vi "WriteIgorDataFile_DP_ver1.0.vi"(2 "2D Data Array In":dbl[][](array[numeric]), 3 "Title Name Array":string[](array[string]), 4 "error in":errorcluster, 5 "Run Info. Comment":string, 7 "file path":path) -> (0 "error out":errorcluster)   [LabVIEW 2012]
doc: "Input 2D data array and Data Save Info. Then, save all the data and info. in Igor format. If \"Title Name Array\" is empty, the title name in igor file would be the title name column from \"Instrs configs 2D arrary\""
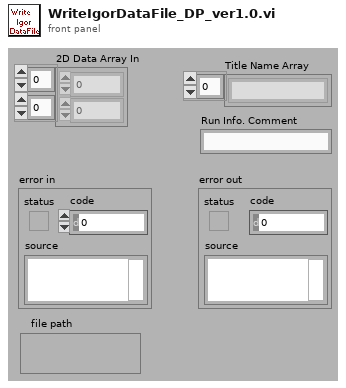
[diagram p1: front panel]
types:
  T1 = enum16{"open", "open or create", "create or replace", "create", "open (read only)"}
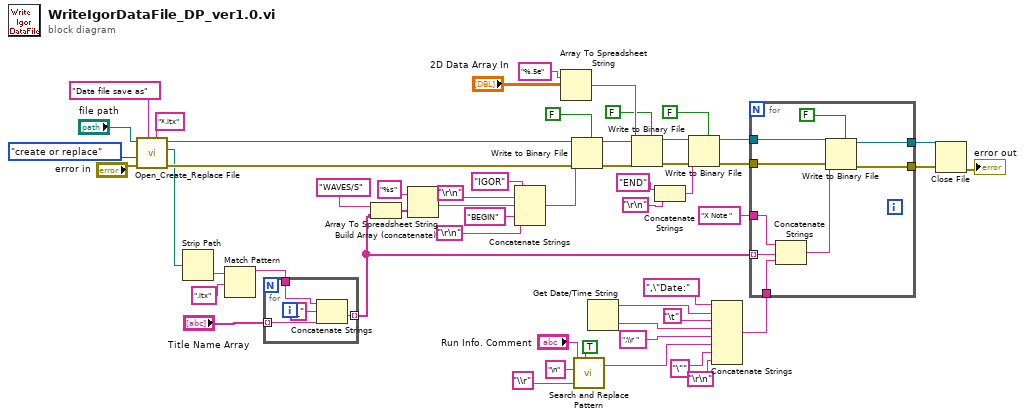
[diagram p0: block diagram]
diagram:
  n1 = call <vilib>:"Open_Create_Replace File.vi"("pattern"="*.itx", "prompt"="Data file save as", "error in (no error)"="error in", "function (open:0)"=T1."create or replace", "file path"="file path") -> ("error out"=w36:errorcluster, "new file path"=w5:path, "refnum"=w35:refnum<file>)  [unwired: 2 in, 2 out]
  n2 = Strip Path(path=w5) -> (name=w8:string)  [unwired: 1 out]
  n3 = Match Pattern(string=w8, regular expression=".itx") -> (before substring=w6:string)  [unwired: 4 out]
  n4 = for {
    tunnel: "Title Name Array" -> [w58] mode=indexing
    tunnel: [w57] -> w24 mode=indexing
    tunnel: w6 -> [w56]
    n5 = Concatenate Strings(w56, "_" ("string"), w58) -> (w57:string)
  }
  n6 = Build Array (concatenate)("WAVES/S", w24) -> (w46:string[])
  n7 = Array To Spreadsheet String(array=w46, 3:"%s" ("format string")) -> (spreadsheet string=w49:string)  [unwired: 1 out]
  n8 = Concatenate Strings("IGOR", "\r\n", w49, "BEGIN", "\r\n") -> (w50:string)
  n9 = Array To Spreadsheet String(array="2D Data Array In", 3:"%.5e" ("format string")) -> (spreadsheet string=w43:string)  [unwired: 1 out]
  n10 = Write to Binary File(file (use dialog)=w35, data=w50, error in=w36, 5:FALSE ("prepend array or string size? (T)")) -> (refnum out=w53:refnum<file>, error out=w54:errorcluster)  [unwired: 3 out]
  n11 = call <vilib>:"Search and Replace Pattern.vi"("string"="Run Info. Comment", "regular expression (\"\")"="\n" ("regular expression (\"\")"), "replace string (\"\")"="\\r", "replace all? (F)"=TRUE) -> ("result string"=w12:string)  [unwired: 2 out]
  n12 = Get Date/Time String() -> (date string=w32:string, time string=w30:string)  [unwired: 3 out]
  n13 = Write to Binary File(file (use dialog)=w53, data=w43, error in=w54, 5:FALSE ("prepend array or string size? (T)")) -> (refnum out=w42:refnum<file>, error out=w41:errorcluster)  [unwired: 3 out]
  n14 = Concatenate Strings("END", "\r\n") -> (w25:string)
  n15 = Write to Binary File(file (use dialog)=w42, data=w25, error in=w41, 5:FALSE ("prepend array or string size? (T)")) -> (refnum out=w21:refnum<file>, error out=w20:errorcluster)  [unwired: 3 out]
  n16 = Concatenate Strings(",\"Date:" ("string"), w32, "\t", w30, ";\\r ", w12, "\"", "\r\n") -> (w16:string)
  n17 = for {
    tunnel: w24 -> [w62] mode=indexing
    tunnel: w21 -> [w66]
    tunnel: w20 -> [w67]
    tunnel: [w65] -> w19
    tunnel: [w64] -> w18
    tunnel: "X Note " -> [w63]
    tunnel: w16 -> [w61]
    n18 = Concatenate Strings(w63, w62, w61) -> (w60:string)
    n19 = Write to Binary File(file (use dialog)=w66, data=w60, error in=w67, 5:FALSE ("prepend array or string size? (T)")) -> (refnum out=w65:refnum<file>, error out=w64:errorcluster)  [unwired: 3 out]
  }
  n20 = Close File(refnum=w19, error in=w18) -> (error out=→"error out":errorcluster)  [unwired: 1 out]
